vi "Day 11.vi"() -> ()   [LabVIEW 2021]
panel:
  out "input":string
  out "input file":path
  out "ouptut 2":u64
  in  "Run [T]/ Example[F]":bool
  out "ouptut 1":u32
  # "Advent of Code 2021 - Day 11 - Dumbo Octopus"
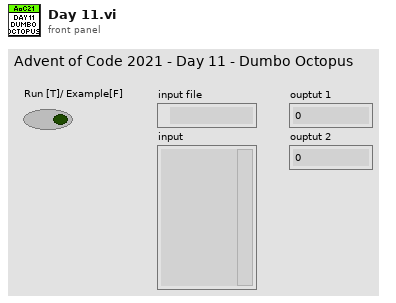
[diagram p1: front panel]
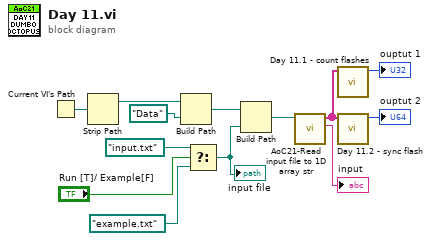
[diagram p0: block diagram]
diagram:
  n1 = Current VI's Path() -> (path=w13:path)
  n2 = Strip Path(path=w13) -> (stripped path=w12:path)  [unwired: 1 out]
  n3 = Build Path(base path=w12, name or relative path=path "Data") -> (appended path=w10:path)
  n4 = Select(t=path "input.txt" ("name or relative path"), s="Run [T]/ Example[F]", f=path "example.txt" ("name or relative path")) -> (s? t:f=w6:path)
  "input file" <- w6
  n5 = Build Path(base path=w10, name or relative path=w6) -> (appended path=w4:path)
  n6 = call "AoC21-Read input file to 1D array str.vi"("input file"=w4) -> ("input text"=→"input":string, "input"=w2:string[])  [unwired: 9 in]
  n7 = call "Day 11.1 - count flashes.vi"("input"=w2) -> ("output"=→"ouptut 1":i32)  [unwired: 10 in]
  n8 = call "Day 11.2 - sync flash.vi"("input"=w2) -> ("output"=→"ouptut 2":i32)  [unwired: 10 in]
